vi "MultiLoop(Queue).vi"() -> ()   [LabVIEW 2023]
panel:
  out "Waveform Chart 4":dbl(graph)
  out "Waveform Chart 5":dbl(graph)
  out "# elements in queue 2":i32
  in  "Stop Button 2":bool
  out "Waveform Chart 3":dbl(graph)
  out "# elements in queue":i32
  out "Waveform Chart 2":dbl(graph)
  in  "Stop Button":bool
  out "Waveform Chart":dbl(graph)
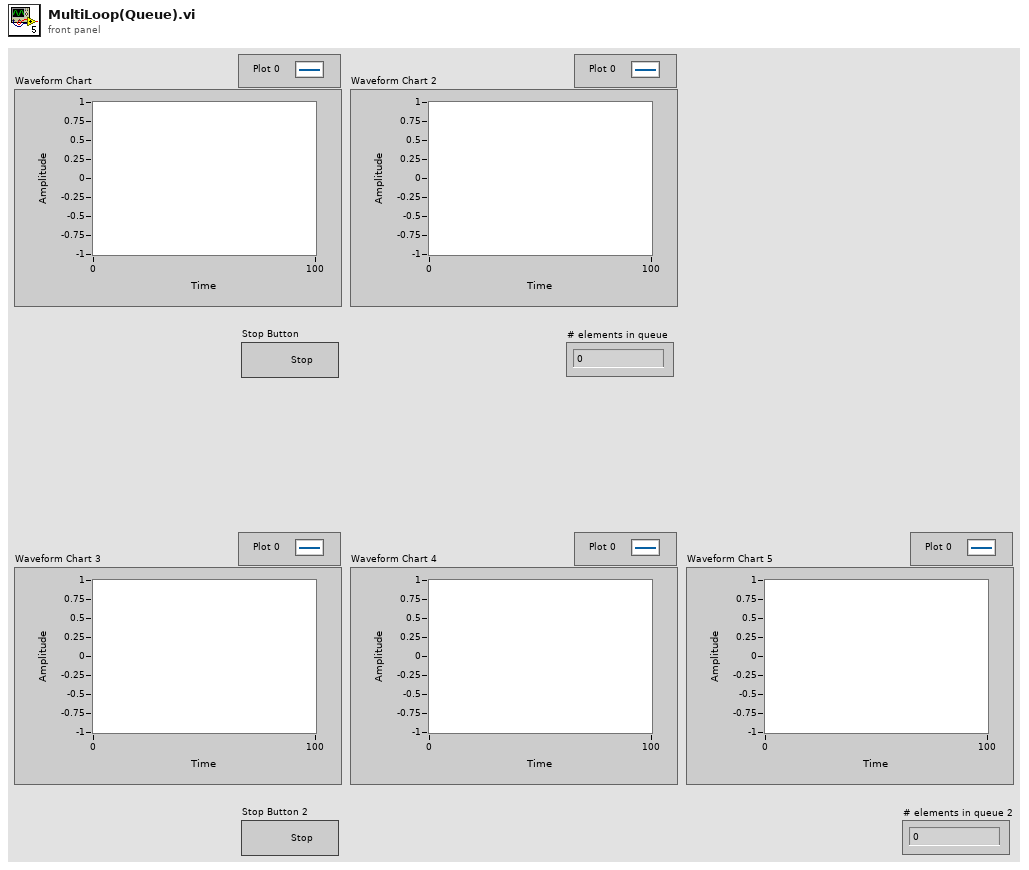
[diagram p1: front panel]
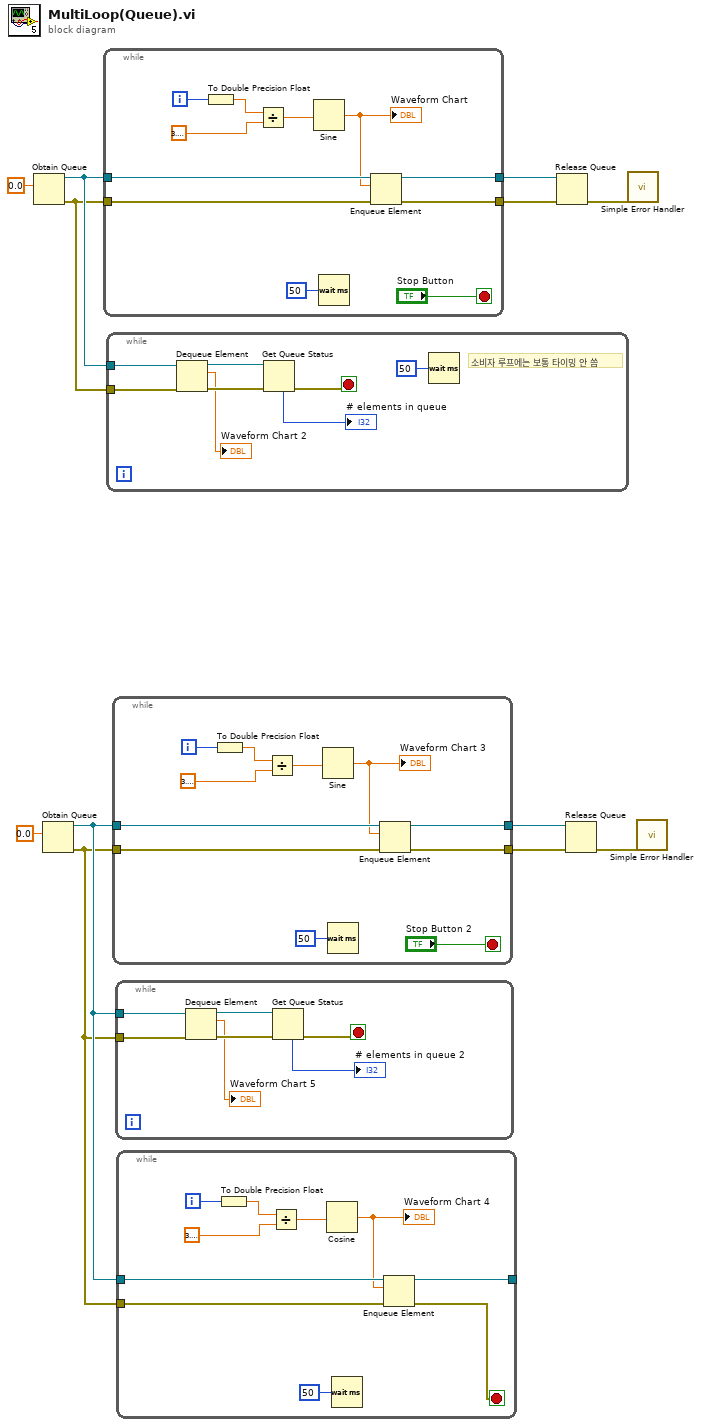
[diagram p0: block diagram]
diagram:
  n1 = Obtain Queue(element data type=0.0) -> (queue out=w8:refnum<queue>, error out=w7:errorcluster)  [unwired: 4 in, 1 out]
  n2 = Obtain Queue(element data type=0.0) -> (queue out=w2:refnum<queue>, error out=w1:errorcluster)  [unwired: 4 in, 1 out]
  n3 = while {
    tunnel: [w17] -> w10
    tunnel: w7 -> [w16]
    tunnel: w8 -> [w15]
    tunnel: [w14] -> w9
    i -> [w23]
    stop <- "Stop Button" stop-if-true
    n4 = To Double Precision Float(number=w23) -> (double precision float=w22:dbl)
    n5 = Divide(x=w22, y=3.141592653589793) -> (x/y=w18:dbl)
    n6 = Sine(x=w18) -> (sin(x)=w13:dbl)
    "Waveform Chart" <- w13
    n7 = Wait (ms)(milliseconds to wait=u32 50) -> ()  [unwired: 1 out]
    n8 = Enqueue Element(queue=w15, element=w13, error in (no error)=w16) -> (queue out=w14:refnum<queue>, error out=w17:errorcluster)  [unwired: 1 in, 1 out]
  }
  n9 = while {
    tunnel: w8 -> [w31]
    tunnel: w7 -> [w29]
    stop <- w27 stop-if-true
    # "소비자 루프에는 보통 타이밍 안 씀"
    n10 = Dequeue Element(queue=w31, error in (no error)=w29) -> (queue out=w30:refnum<queue>, element=→"Waveform Chart 2":dbl, error out=w28:errorcluster)  [unwired: 1 in, 1 out]
    n11 = Get Queue Status(queue=w30, error in (no error)=w28) -> (error out=w27:errorcluster, # elements in queue=→"# elements in queue":i32)  [unwired: 1 in, 6 out]
    n12 = Wait (ms)(milliseconds to wait=u32 50) -> ()  [unwired: 1 out]
  }
  n13 = while {
    tunnel: [w36] -> w4
    tunnel: w1 -> [w35]
    tunnel: w2 -> [w34]
    tunnel: [w33] -> w3
    i -> [w42]
    stop <- "Stop Button 2" stop-if-true
    n14 = To Double Precision Float(number=w42) -> (double precision float=w41:dbl)
    n15 = Divide(x=w41, y=3.141592653589793) -> (x/y=w37:dbl)
    n16 = Sine(x=w37) -> (sin(x)=w32:dbl)
    "Waveform Chart 3" <- w32
    n17 = Wait (ms)(milliseconds to wait=u32 50) -> ()  [unwired: 1 out]
    n18 = Enqueue Element(queue=w34, element=w32, error in (no error)=w35) -> (queue out=w33:refnum<queue>, error out=w36:errorcluster)  [unwired: 1 in, 1 out]
  }
  n19 = while {
    tunnel: w2 -> [w49]
    tunnel: w1 -> [w47]
    stop <- w45 stop-if-true
    n20 = Dequeue Element(queue=w49, error in (no error)=w47) -> (queue out=w48:refnum<queue>, element=→"Waveform Chart 5":dbl, error out=w46:errorcluster)  [unwired: 1 in, 1 out]
    n21 = Get Queue Status(queue=w48, error in (no error)=w46) -> (error out=w45:errorcluster, # elements in queue=→"# elements in queue 2":i32)  [unwired: 1 in, 6 out]
  }
  n22 = while {
    tunnel: w1 -> [w54]
    tunnel: w2 -> [w53]
    tunnel: [w52] -> _
    i -> [w59]
    stop <- w50 stop-if-true
    n23 = To Double Precision Float(number=w59) -> (double precision float=w58:dbl)
    n24 = Divide(x=w58, y=3.141592653589793) -> (x/y=w55:dbl)
    n25 = Cosine(x=w55) -> (cos(x)=w51:dbl)
    "Waveform Chart 4" <- w51
    n26 = Wait (ms)(milliseconds to wait=u32 50) -> ()  [unwired: 1 out]
    n27 = Enqueue Element(queue=w53, element=w51, error in (no error)=w54) -> (queue out=w52:refnum<queue>, error out=w50:errorcluster)  [unwired: 1 in, 1 out]
  }
  n28 = Release Queue(queue=w9, error in (no error)=w10) -> (error out=w11:errorcluster)  [unwired: 1 in, 2 out]
  n29 = Release Queue(queue=w3, error in (no error)=w4) -> (error out=w5:errorcluster)  [unwired: 1 in, 2 out]
  n30 = call <vilib>:"Simple Error Handler.vi"("error in (no error)"=w11) -> ()  [unwired: 4 in, 5 out]
  n31 = call <vilib>:"Simple Error Handler.vi"("error in (no error)"=w5) -> ()  [unwired: 4 in, 5 out]
